vi "Cleanup.vi"(8 "error in (no error)":errorcluster, 11 "Deck in":refnum<class "Sample.lvclass">) -> (0 "error out":errorcluster, 3 "Deck out":refnum<class "Sample.lvclass">)   [LabVIEW 2020, in "Sample.lvclass"]
uses:
  Sample.lvclass
  Sample.lvclass/Sample.ctl
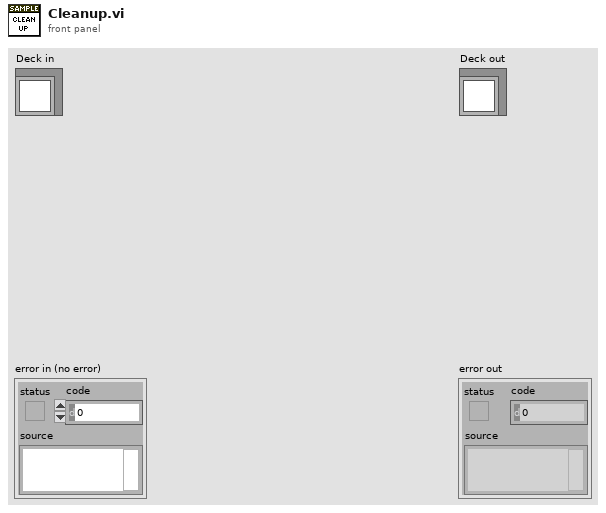
[diagram p1: front panel]
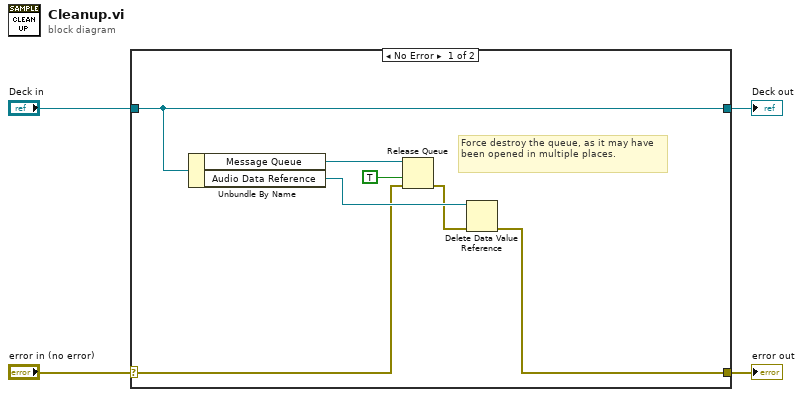
[diagram p0: block diagram]
diagram:
  n1 = case shown="No Error" "error in (no error)" {
    selector: "error in (no error)" -> [w6 w13]
    tunnel: [w5 w13] -> w3
    tunnel: [w11 w12] -> w1
    tunnel: "Deck in" -> [w11 w12]
    frame No Error {
      # "Force destroy the queue, as it may have been opened in multiple places."
      n2 = Unbundle By Name(w11) -> ("Message Queue"=w10:refnum<queue>, "Audio Data Reference"=w8:refnum<data-value>)
      n3 = Release Queue(queue=w10, force destroy? (F)=TRUE, error in (no error)=w6) -> (error out=w7:errorcluster)  [unwired: 2 out]
      n4 = Delete Data Value Reference(data value reference=w8, error in=w7) -> (error out=w5:errorcluster)  [unwired: 1 out]
    }
    frame Error {
    }
  }
  "error out" <- w3
  "Deck out" <- w1
